vi "DiffDrivePoseEst2_InterpRecord_New.vi"(8 "RightDistance":dbl, 9 "LeftDistance":dbl, 10 "GyroAngle":T3 {"SIN" format="%13.4f"; "COS" format="%13.4f"; "VALUE" format="%13.4f"}, 11 "M_POSE_Meters":T1 {"ROTATION"."SIN" format="%13.4f"; "ROTATION"."COS" format="%13.4f"; "ROTATION"."VALUE" format="%13.4f"; "TRANSLATION"."Y" format="%14.3f"; "TRANSLATION"."X" format="%14.3f"}) -> (3 "DIFF_DRIVE_POSE_EST2_INTERP_RECORD":T4 {"GyroAngle"."SIN" format="%13.4f"; "GyroAngle"."COS" format="%13.4f"; "GyroAngle"."VALUE" format="%13.4f"; "PoseMeters"."ROTATION"."SIN" format="%13.4f"; "PoseMeters"."ROTATION"."COS" format="%13.4f"; "PoseMeters"."ROTATION"."VALUE" format="%13.4f"; "PoseMeters"."TRANSLATION"."Y" format="%14.3f"; "PoseMeters"."TRANSLATION"."X" format="%14.3f"})   [LabVIEW 2019, in "Trajectory_Library.lvlib"]
uses:
  Trajectory_Library.lvlib
  TypeDef/DIFF_DRIVE_POSE_EST2_INTERP_RECORD.ctl
  TypeDef/POSE2D.ctl
  TypeDef/TRANSLATION2D.ctl
  TypeDef/ROTATION2D.ctl
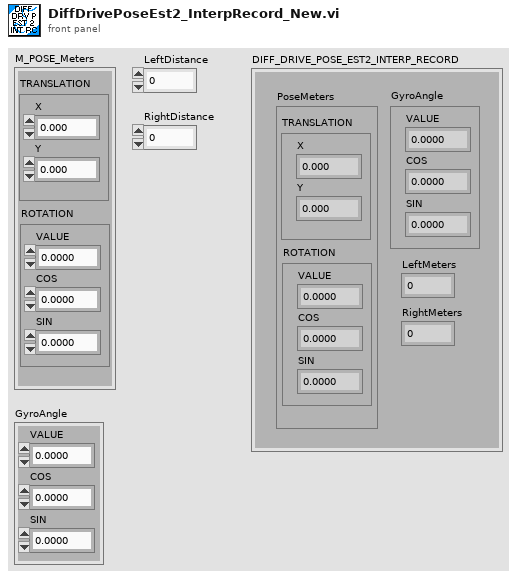
[diagram p1: front panel]
types:
  T1 = typedef "Trajectory_Library.lvlib/POSE2D.ctl" = cluster{"TRANSLATION":T2, "ROTATION":T3}
  T2 = typedef "Trajectory_Library.lvlib/TRANSLATION2D.ctl" = cluster{"X":dbl, "Y":dbl}
  T3 = typedef "Trajectory_Library.lvlib/ROTATION2D.ctl" = cluster{"VALUE":dbl, "COS":dbl, "SIN":dbl}
  T4 = typedef "Trajectory_Library.lvlib/DIFF_DRIVE_POSE_EST2_INTERP_RECORD.ctl" = cluster{"PoseMeters":T1, "GyroAngle":T3, "LeftMeters":dbl, "RightMeters":dbl}
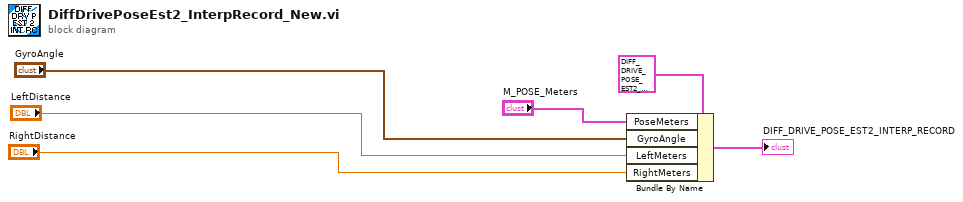
[diagram p0: block diagram]
diagram:
  n1 = Bundle By Name(cluster=T4 {"PoseMeters"={"TRANSLATION"={"X"=0.0, "Y"=0.0}, "ROTATION"={"VALUE"=0.0, "COS"=1.0, "SIN"=0.0}}, "GyroAngle"={"VALUE"=0.0, "COS"=1.0, "SIN"=0.0}, "LeftMeters"=0.0, "RightMeters"=0.0} ("DIFF_DRIVE_POSE_EST2_INTERP_RECORD"), "PoseMeters"="M_POSE_Meters", "GyroAngle"="GyroAngle", "LeftMeters"="LeftDistance", "RightMeters"="RightDistance") -> (→"DIFF_DRIVE_POSE_EST2_INTERP_RECORD":T4)
